vi "set_fp_array.vi"(0 "LstBox Refnum":refnum<vi>, 1 "F Values Array":dbl[][](array[numeric]), 2 "Frekanslar":dbl[](array[numeric]), 3 "frekans index":dbl, 4 "AD F/P Array":dbl[][](array[numeric]), 5 "10R F/P Array":dbl[][](array[numeric]), 6 "1R F/P Array":dbl[][](array[numeric]), 7 "Wagner F/P Array":dbl[][](array[numeric]), 8 "Kelvin F/P Array":dbl[][](array[numeric]), 9 "Direnc 1 - Direnc 2":u16(ring)=2 items=["1M(Ohm) / 100K(Ohm)", "100K(Ohm) / 10K(Ohm)", "10K(Ohm) / 1K(Ohm)", "1K(Ohm) / 100(Ohm)", "100(Ohm) / 10(Ohm)", "10(Ohm) / 1(Ohm)"]) -> (14 "output ad f/p":dbl[][](array[numeric]), 15 "output 10r f/p":dbl[][](array[numeric]), 16 "output 1r f/p":dbl[][](array[numeric]), 17 "output w f/p":dbl[][](array[numeric]), 18 "output k f/p":dbl[][](array[numeric]))   [LabVIEW 2014]
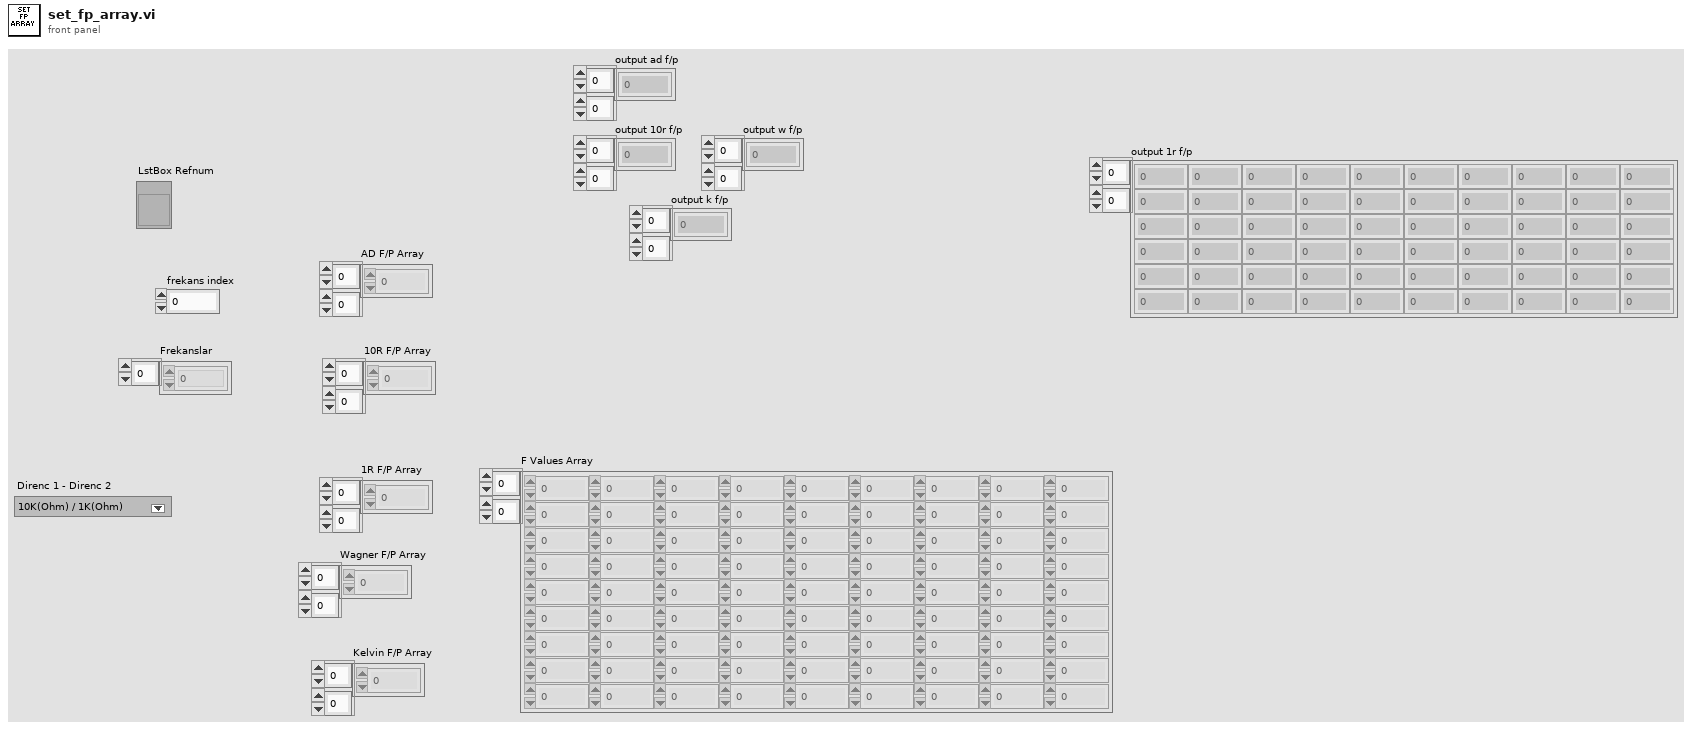
[diagram p1: front panel]
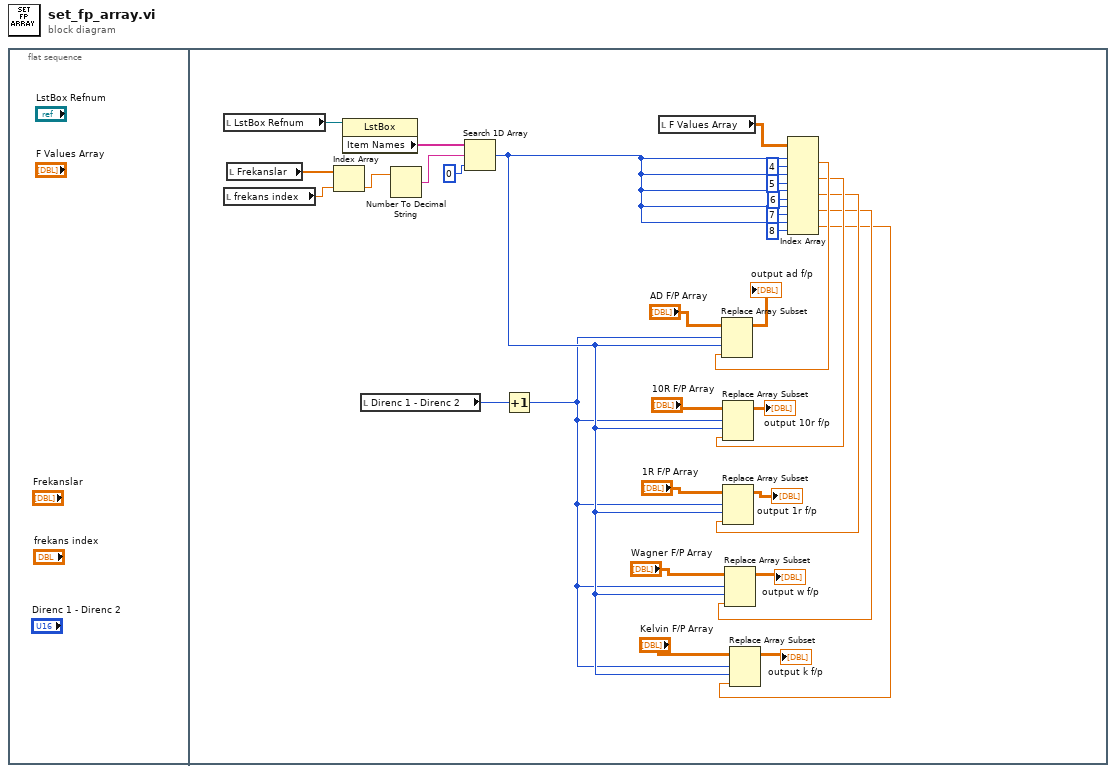
[diagram p0: block diagram]
diagram:
  n1 = flat-sequence {
    frame #0 {
    }
    frame #1 {
      n2 = local read "LstBox Refnum"() -> (w8:refnum<vi>)
      n3 = local read "frekans index"() -> (w6:dbl)
      n4 = local read "Frekanslar"() -> (w7:dbl[])
      n5 = Index Array(array=w7, index=w6) -> (element=w2:dbl)
      n6 = property class="LstBox"(reference=w8) -> ("Item Names"=w5:string[])  [unwired: 1 in, 2 out]
      n7 = local read "Direnc 1 - Direnc 2"() -> (w3:u16)
      n8 = Number To Decimal String(number=w2) -> (decimal integer string=w1:string)  [unwired: 1 in]
      n9 = Search 1D Array(1D array=w5, element=w1, start index (0)=0) -> (index of element=w30:i32)
      n10 = Increment(x=w3) -> (x+1=w19:u16)
      n11 = local read "F Values Array"() -> (w31:dbl[][])
      n12 = Index Array(array=w31, index (row) #1=w30, index (col) #1=4 ("disabled index (col)"), index (row) #2=w30, index (col) #2=5 ("disabled index (col)"), index (row) #3=w30, index (col) #3=6 ("disabled index (col)"), index (row) #4=w30, index (col) #4=7 ("disabled index (col)"), index (row) #5=w30, index (col) #5=8 ("disabled index (col)")) -> (element #1=w18:dbl, element #2=w17:dbl, element #3=w16:dbl, element #4=w15:dbl, element #5=w14:dbl)
      n13 = Replace Array Subset(array="AD F/P Array", new element=w18, index (row)=w19, index (col)=w30) -> (→"output ad f/p":dbl[][])
      n14 = Replace Array Subset(array="10R F/P Array", new element=w17, index (row)=w19, index (col)=w30) -> (→"output 10r f/p":dbl[][])
      n15 = Replace Array Subset(array="1R F/P Array", new element=w16, index (row)=w19, index (col)=w30) -> (→"output 1r f/p":dbl[][])
      n16 = Replace Array Subset(array="Wagner F/P Array", new element=w15, index (row)=w19, index (col)=w30) -> (→"output w f/p":dbl[][])
      n17 = Replace Array Subset(array="Kelvin F/P Array", new element=w14, index (row)=w19, index (col)=w30) -> (→"output k f/p":dbl[][])
    }
  }
